vi "mupRelease.vi"(8 "error in (no error)":errorcluster, 11 "hParser in":u64) -> (0 "error out":errorcluster)   [LabVIEW 2015, in "mupLib.lvlib"]
doc: "Close the muParser instance."
uses:
  mupLib.lvlib
  libmuparser-lv.dll
panel:
  # "Close the muParser instance."
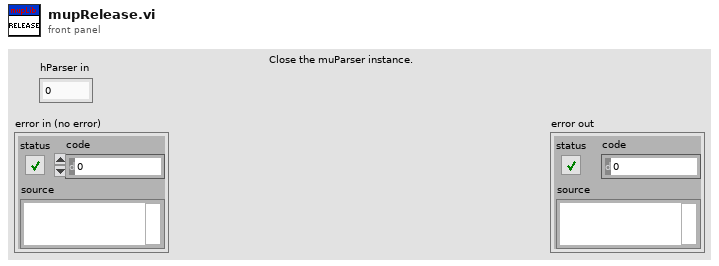
[diagram p1: front panel]
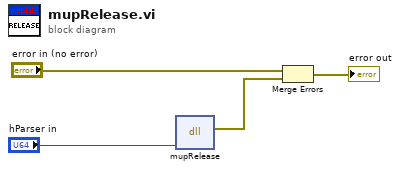
[diagram p0: block diagram]
diagram:
  n1 = dll-call lib="C:/Users/leonidas/Documents/GitHub/LV-muParser/mupLib/libmuparser-lv.dll" fn="mupRelease"("hParser"="hParser in") -> (error out=w3:errorcluster)  [unwired: 5 in, 1 out]
  n2 = Merge Errors("error in (no error)", w3) -> (→"error out":errorcluster)
